vi "wechatSuperResolutionCoffeeModel.vi"() -> (0 "Model":string, 1 "ProtoTxt":string)   [LabVIEW 2020]
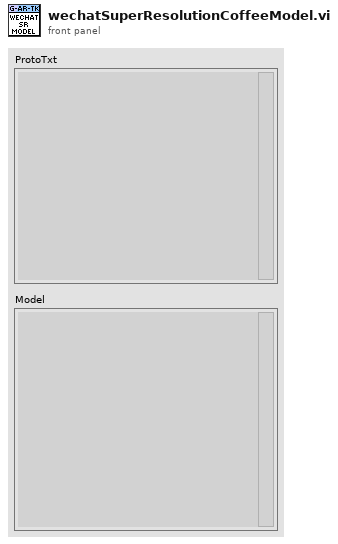
[diagram p1: front panel]
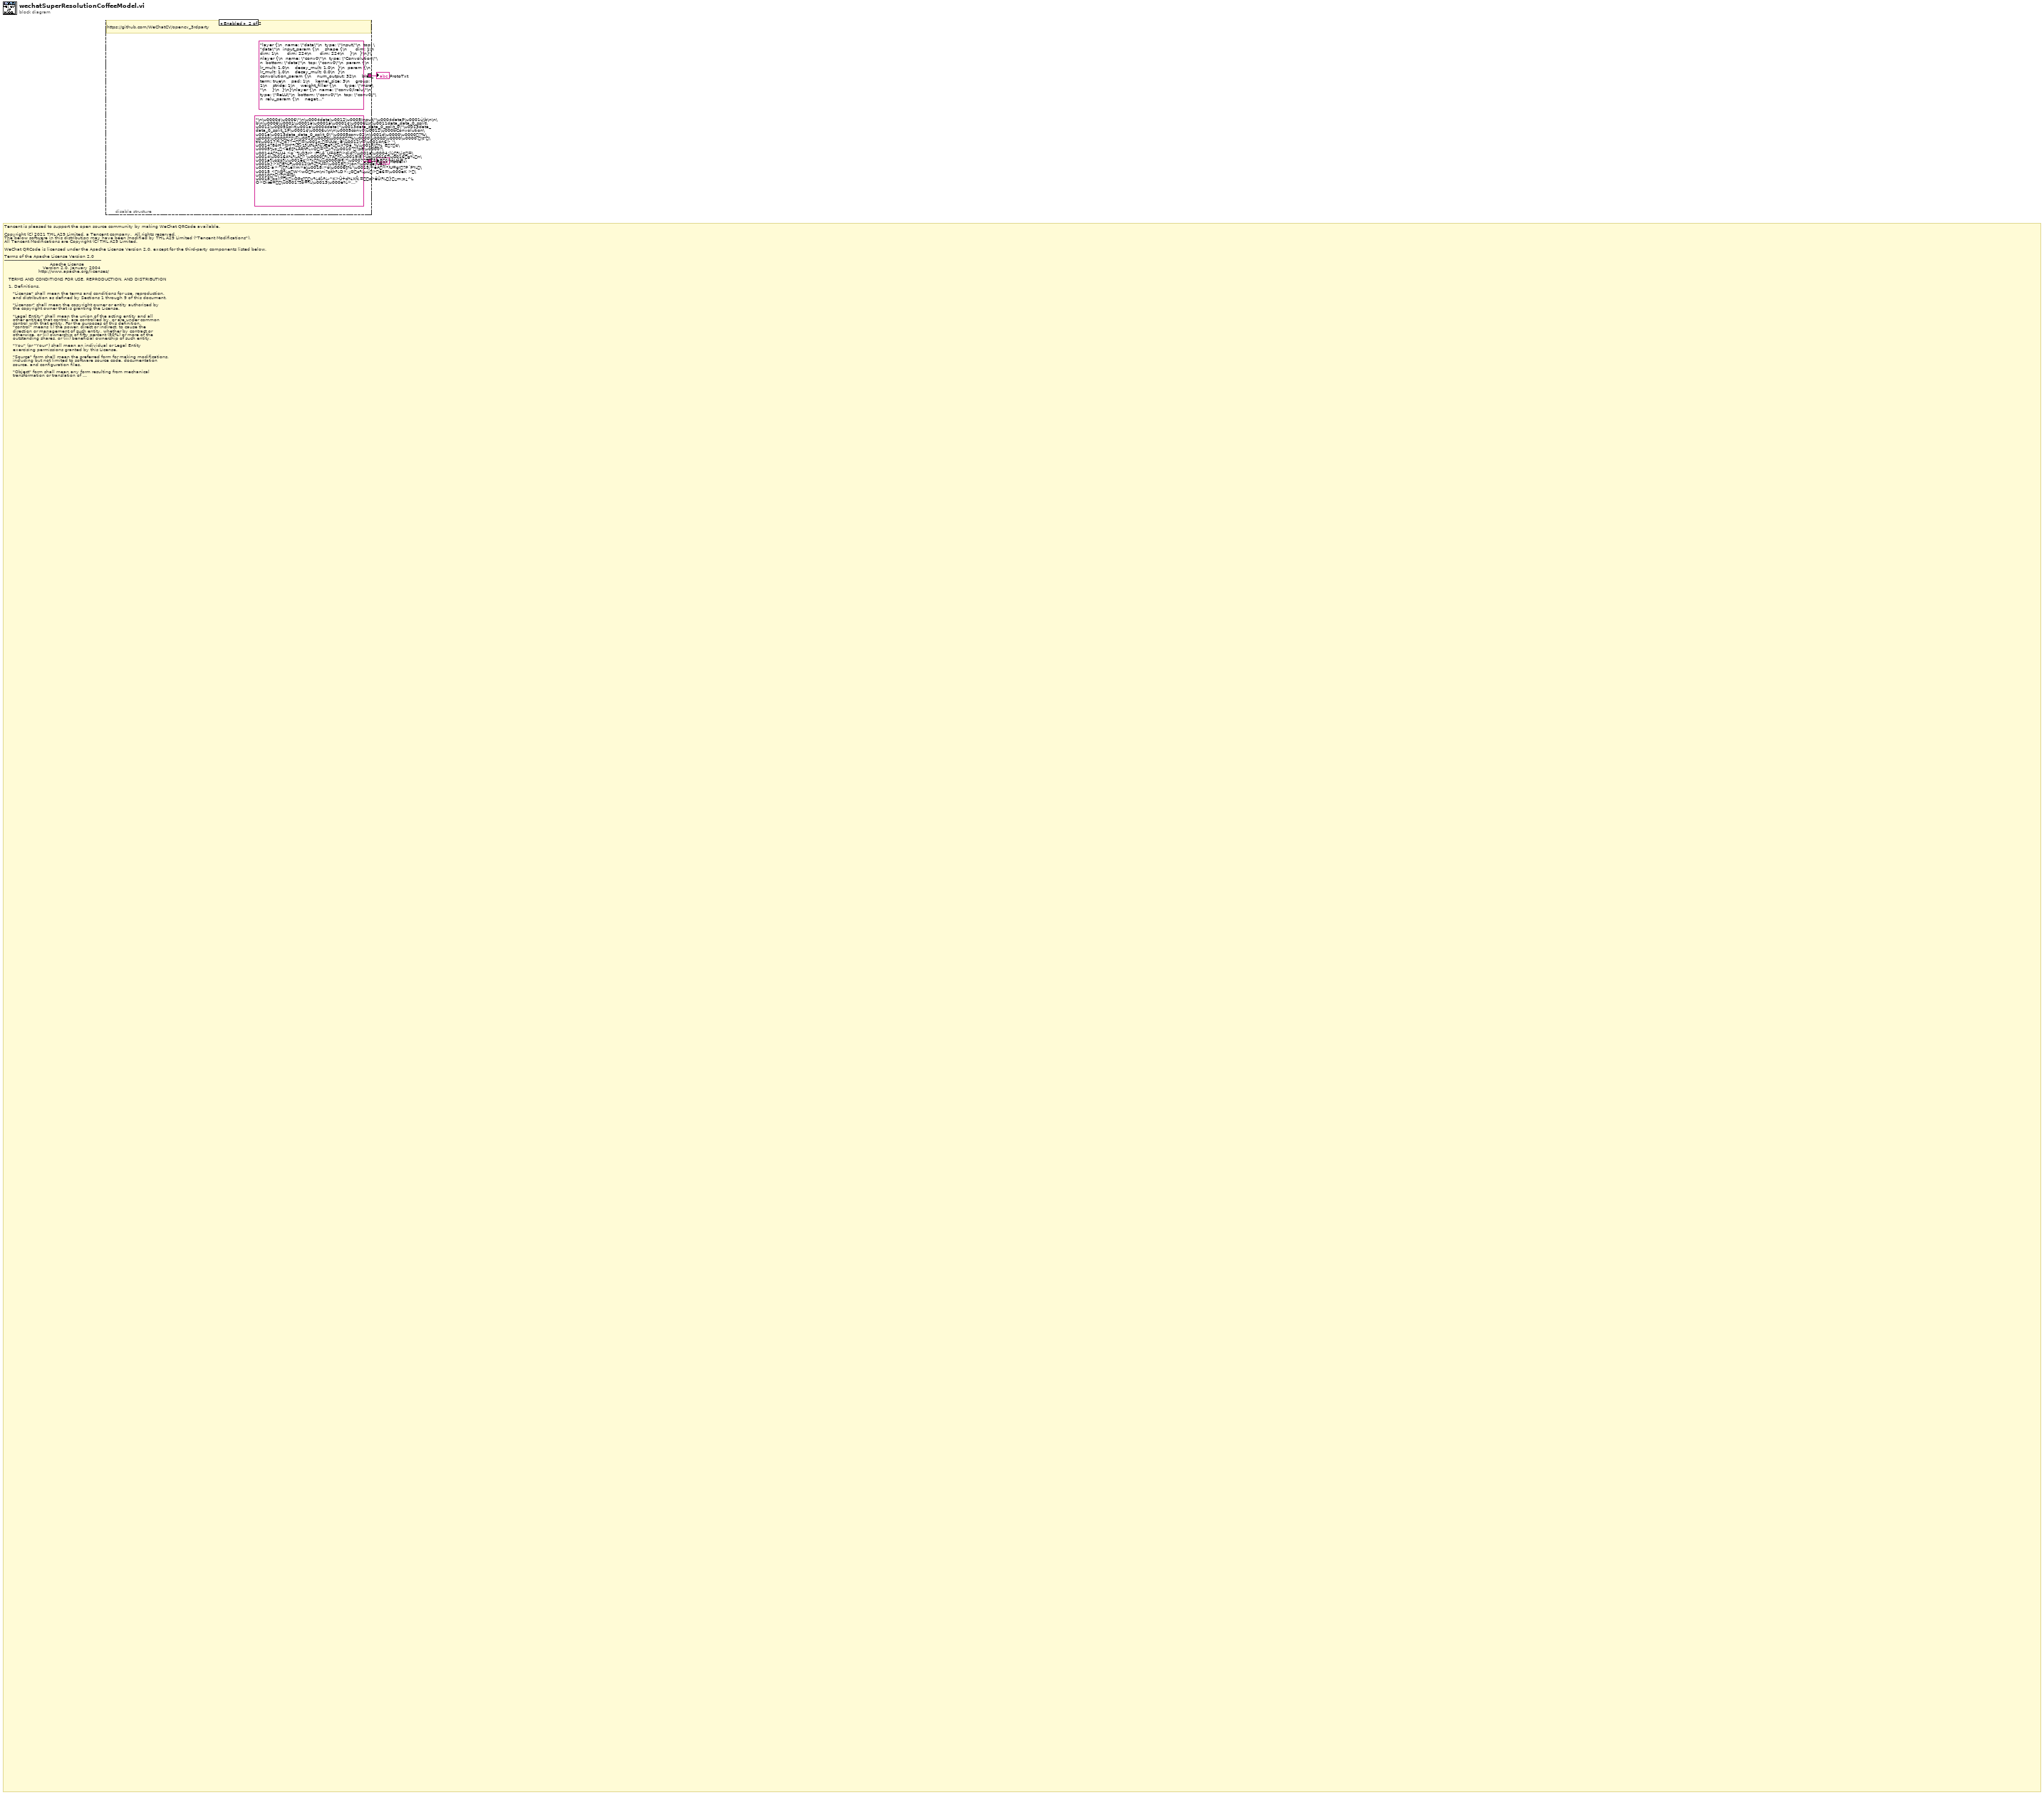
[diagram p0: block diagram]
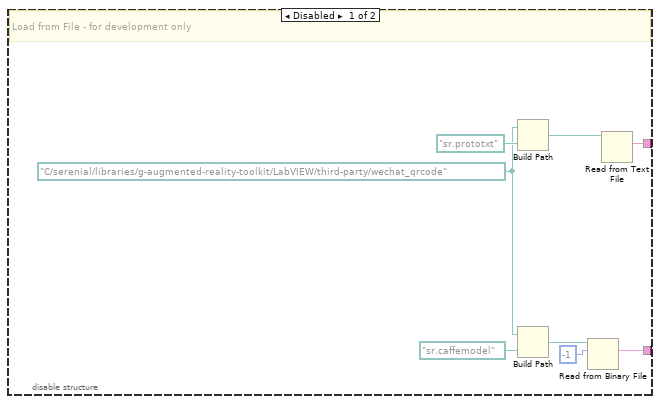
[diagram p2: hidden frame]
diagram:
  # "Tencent is pleased to support the open source community by making WeChat QRCode available.\n\nCopyright (C) 2021 THL A29 Limited, a Tencent company.  All rights reserved.\nThe below software in this distribution may have been modified by THL A29 Limited (\"Tencent Modifications\").\nAll Tencent Modifications are Copyright (C) THL A29 Limited.\n\nWeChat QRCode is licensed under the Apache License Version 2.0, except for the third-party components listed below.\n\nTerms of the Apache License Version 2.0\n--------------------------------------------------------------------\n                                Apache License\n                           Version 2.0, January 2004\n                        http://www.apache.org/licenses/\n\n   TERMS AND CONDITIONS FOR USE, REPRODUCTION, AND DISTRIBUTION\n\n   1. Definitions.\n\n      \"License\" shall mean the terms and conditions for use, reproduction,\n      and distribution as defined by Sections 1 through 9 of this document.\n\n      \"Licensor\" shall mean the copyright owner or entity authorized by\n      the copyright owner that is granting the License.\n\n      \"Legal Entity\" shall mean the union of the acting entity and all\n      other entities that control, are controlled by, or are under common\n      control with that entity. For the purposes of this definition,\n      \"control\" means (i) the power, direct or indirect, to cause the\n      direction or management of such entity, whether by contract or\n      otherwise, or (ii) ownership of fifty percent (50%) or more of the\n      outstanding shares, or (iii) beneficial ownership of such entity.\n\n      \"You\" (or \"Your\") shall mean an individual or Legal Entity\n      exercising permissions granted by this License.\n\n      \"Source\" form shall mean the preferred form for making modifications,\n      including but not limited to software source code, documentation\n      source, and configuration files.\n\n      \"Object\" form shall mean any form resulting from mechanical\n      transformation or translation of a Source form, including but\n      not limited to compiled object code, generated documentation,\n      and conversions to other media types.\n\n      \"Work\" shall mean the work of authorship, whether in Source or\n      Object form, made available under the License, as indicated by a\n      copyright notice that is included in or attached to the work\n      (an example is provided in the Appendix below).\n\n      \"Derivative Works\" shall mean any work, whether in Source or Object\n      form, that is based on (or derived from) the Work and for which the\n      editorial revisions, annotations, elaborations, or other modifications\n      represent, as a whole, an original work of authorship. For the purposes\n      of this License, Derivative Works shall not include works that remain\n      separable from, or merely link (or bind by name) to the interfaces of,\n      the Work and Derivative Works thereof.\n\n      \"Contribution\" shall mean any work of authorship, including\n      the original version of the Work and any modifications or additions\n      to that Work or Derivative Works thereof, that is intentionally\n      submitted to Licensor for inclusion in the Work by the copyright owner\n      or by an individual or Legal Entity authorized to submit on behalf of\n      the copyright owner. For the purposes of this definition, \"submitted\"\n      means any form of electronic, verbal, or written communication sent\n      to the Licensor or its representatives, including but not limited to\n      communication on electronic mailing lists, source code control systems,\n      and issue tracking systems that are managed by, or on behalf of, the\n      Licensor for the purpose of discussing and improving the Work, but\n      excluding communication that is conspicuously marked or otherwise\n      designated in writing by the copyright owner as \"Not a Contribution.\"\n\n      \"Contributor\" shall mean Licensor and any individual or Legal Entity\n      on behalf of whom a Contribution has been received by Licensor and\n      subsequently incorporated within the Work.\n\n   2. Grant of Copyright License. Subject to the terms and conditions of\n      this License, each Contributor hereby grants to You a perpetual,\n      worldwide, non-exclusive, no-charge, royalty-free, irrevocable\n      copyright license to reproduce, prepare Derivative Works of,\n      publicly display, publicly perform, sublicense, and distribute the\n      Work and such Derivative Works in Source or Object form.\n\n   3. Grant of Patent License. Subject to the terms and conditions of\n      this License, each Contributor hereby grants to You a perpetual,\n      worldwide, non-exclusive, no-charge, royalty-free, irrevocable\n      (except as stated in this section) patent license to make, have made,\n      use, offer to sell, sell, import, and otherwise transfer the Work,\n      where such license applies only to those patent claims licensable\n      by such Contributor that are necessarily infringed by their\n      Contribution(s) alone or by combination of their Contribution(s)\n      with the Work to which such Contribution(s) was submitted. If You\n      institute patent litigation against any entity (including a\n      cross-claim or counterclaim in a lawsuit) alleging that the Work\n      or a Contribution incorporated within the Work constitutes direct\n      or contributory patent infringement, then any patent licenses\n      granted to You under this License for that Work shall terminate\n      as of the date such litigation is filed.\n\n   4. Redistribution. You may reproduce and distribute copies of the\n      Work or Derivative Works thereof in any medium, with or without\n      modifications, and in Source or Object form, provided that You\n      meet the following conditions:\n\n      (a) You must give any other recipients of the Work or\n          Derivative Works a copy of this License; and\n\n      (b) You must cause any modified files to carry prominent notices\n          stating that You changed the files; and\n\n      (c) You must retain, in the Source form of any Derivative Works\n          that You distribute, all copyright, patent, trademark, and\n          attribution notices from the Source form of the Work,\n          excluding those notices that do not pertain to any part of\n          the Derivative Works; and\n\n      (d) If the Work includes a \"NOTICE\" text file as part of its\n          distribution, then any Derivative Works that You distribute must\n          include a readable copy of the attribution notices contained\n          within such NOTICE file, excluding those notices that do not\n          pertain to any part of the Derivative Works, in at least one\n          of the following places: within a NOTICE text file distributed\n          as part of the Derivative Works; within the Source form or\n          documentation, if provided along with the Derivative Works; or,\n          within a display generated by the Derivative Works, if and\n          wherever such third-party notices normally appear. The contents\n          of the NOTICE file are for informational purposes only and\n          do not modify the License. You may add Your own attribution\n          notices within Derivative Works that You distribute, alongside\n          or as an addendum to the NOTICE text from the Work, provided\n          that such additional attribution notices cannot be construed\n          as modifying the License.\n\n      You may add Your own copyright statement to Your modifications and\n      may provide additional or different license terms and conditions\n      for use, reproduction, or distribution of Your modifications, or\n      for any such Derivative Works as a whole, provided Your use,\n      reproduction, and distribution of the Work otherwise complies with\n      the conditions stated in this License.\n\n   5. Submission of Contributions. Unless You explicitly state otherwise,\n      any Contribution intentionally submitted for inclusion in the Work\n      by You to the Licensor shall be under the terms and conditions of\n      this License, without any additional terms or conditions.\n      Notwithstanding the above, nothing herein shall supersede or modify\n      the terms of any separate license agreement you may have executed\n      with Licensor regarding such Contributions.\n\n   6. Trademarks. This License does not grant permission to use the trade\n      names, trademarks, service marks, or product names of the Licensor,\n      except as required for reasonable and customary use in describing the\n      origin of the Work and reproducing the content of the NOTICE file.\n\n   7. Disclaimer of Warranty. Unless required by applicable law or\n      agreed to in writing, Licensor provides the Work (and each\n      Contributor provides its Contributions) on an \"AS IS\" BASIS,\n      WITHOUT WARRANTIES OR CONDITIONS OF ANY KIND, either express or\n      implied, including, without limitation, any warranties or conditions\n      of TITLE, NON-INFRINGEMENT, MERCHANTABILITY, or FITNESS FOR A\n      PARTICULAR PURPOSE. You are solely responsible for determining the\n      appropriateness of using or redistributing the Work and assume any\n      risks associated with Your exercise of permissions under this License.\n\n   8. Limitation of Liability. In no event and under no legal theory,\n      whether in tort (including negligence), contract, or otherwise,\n      unless required by applicable law (such as deliberate and grossly\n      negligent acts) or agreed to in writing, shall any Contributor be\n      liable to You for damages, including any direct, indirect, special,\n      incidental, or consequential damages of any character arising as a\n      result of this License or out of the use or inability to use the\n      Work (including but not limited to damages for loss of goodwill,\n      work stoppage, computer failure or malfunction, or any and all\n      other commercial damages or losses), even if such Contributor\n      has been advised of the possibility of such damages.\n\n   9. Accepting Warranty or Additional Liability. While redistributing\n      the Work or Derivative Works thereof, You may choose to offer,\n      and charge a fee for, acceptance of support, warranty, indemnity,\n      or other liability obligations and/or rights consistent with this\n      License. However, in accepting such obligations, You may act only\n      on Your own behalf and on Your sole responsibility, not on behalf\n      of any other Contributor, and only if You agree to indemnify,\n      defend, and hold each Contributor harmless for any liability\n      incurred by, or claims asserted against, such Contributor by reason\n      of your accepting any such warranty or additional liability.\n\nEND OF TERMS AND CONDITIONS\n\n\n\nOther dependencies and licenses:\n\nOpen Source Software Licensed under the Apache License Version 2.0:\n--------------------------------------------------------------------\n1. zxing\nCopyright (c) zxing authors and contributors\nPlease note this software may have been modified by Tencent.\n\nTerms of the Apache License Version 2.0:\n--------------------------------------------------------------------\nApache License\n\nVersion 2.0, January 2004\n\nhttp://www.apache.org/licenses/\n\nTERMS AND CONDITIONS FOR USE, REPRODUCTION, AND DISTRIBUTION\n\n1. Definitions.\n\n\"License\" shall mean the terms and conditions for use, reproduction, and distribution as defined by Sections 1 through 9 of this document.\n\n\"Licensor\" shall mean the copyright owner or entity authorized by the copyright owner that is granting the License.\n\n\"Legal Entity\" shall mean the union of the acting entity and all other entities that control, are controlled by, or are under common control with that entity. For the purposes of this definition, \"control\" means (i) the power, direct or indirect, to cause the direction or management of such entity, whether by contract or otherwise, or (ii) ownership of fifty percent (50%) or more of the outstanding shares, or (iii) beneficial ownership of such entity.\n\n\"You\" (or \"Your\") shall mean an individual or Legal Entity exercising permissions granted by this License.\n\n\"Source\" form shall mean the preferred form for making modifications, including but not limited to software source code, documentation source, and configuration files.\n\n\"Object\" form shall mean any form resulting from mechanical transformation or translation of a Source form, including but not limited to compiled object code, generated documentation, and conversions to other media types.\n\n\"Work\" shall mean the work of authorship, whether in Source or Object form, made available under the License, as indicated by a copyright notice that is included in or attached to the work (an example is provided in the Appendix below).\n\n\"Derivative Works\" shall mean any work, whether in Source or Object form, that is based on (or derived from) the Work and for which the editorial revisions, annotations, elaborations, or other modifications represent, as a whole, an original work of authorship. For the purposes of this License, Derivative Works shall not include works that remain separable from, or merely link (or bind by name) to the interfaces of, the Work and Derivative Works thereof.\n\n\"Contribution\" shall mean any work of authorship, including the original version of the Work and any modifications or additions to that Work or Derivative Works thereof, that is intentionally submitted to Licensor for inclusion in the Work by the copyright owner or by an individual or Legal Entity authorized to submit on behalf of the copyright owner. For the purposes of this definition, \"submitted\" means any form of electronic, verbal, or written communication sent to the Licensor or its representatives, including but not limited to communication on electronic mailing lists, source code control systems, and issue tracking systems that are managed by, or on behalf of, the Licensor for the purpose of discussing and improving the Work, but excluding communication that is conspicuously marked or otherwise designated in writing by the copyright owner as \"Not a Contribution.\"\n\n\"Contributor\" shall mean Licensor and any individual or Legal Entity on behalf of whom a Contribution has been received by Licensor and subsequently incorporated within the Work.\n\n2. Grant of Copyright License. Subject to the terms and conditions of this License, each Contributor hereby grants to You a perpetual, worldwide, non-exclusive, no-charge, royalty-free, irrevocable copyright license to reproduce, prepare Derivative Works of, publicly display, publicly perform, sublicense, and distribute the Work and such Derivative Works in Source or Object form.\n\n3. Grant of Patent License. Subject to the terms and conditions of this License, each Contributor hereby grants to You a perpetual, worldwide, non-exclusive, no-charge, royalty-free, irrevocable (except as stated in this section) patent license to make, have made, use, offer to sell, sell, import, and otherwise transfer the Work, where such license applies only to those patent claims licensable by such Contributor that are necessarily infringed by their Contribution(s) alone or by combination of their Contribution(s) with the Work to which such Contribution(s) was submitted. If You institute patent litigation against any entity (including a cross-claim or counterclaim in a lawsuit) alleging that the Work or a Contribution incorporated within the Work constitutes direct or contributory patent infringement, then any patent licenses granted to You under this License for that Work shall terminate as of the date such litigation is filed.\n\n4. Redistribution. You may reproduce and distribute copies of the Work or Derivative Works thereof in any medium, with or without modifications, and in Source or Object form, provided that You meet the following conditions:\n\nYou must give any other recipients of the Work or Derivative Works a copy of this License; and\nYou must cause any modified files to carry prominent notices stating that You changed the files; and\nYou must retain, in the Source form of any Derivative Works that You distribute, all copyright, patent, trademark, and attribution notices from the Source form of the Work, excluding those notices that do not pertain to any part of the Derivative Works; and\nIf the Work includes a \"NOTICE\" text file as part of its distribution, then any Derivative Works that You distribute must include a readable copy of the attribution notices contained within such NOTICE file, excluding those notices that do not pertain to any part of the Derivative Works, in at least one of the following places: within a NOTICE text file distributed as part of the Derivative Works; within the Source form or documentation, if provided along with the Derivative Works; or, within a display generated by the Derivative Works, if and wherever such third-party notices normally appear. The contents of the NOTICE file are for informational purposes only and do not modify the License. You may add Your own attribution notices within Derivative Works that You distribute, alongside or as an addendum to the NOTICE text from the Work, provided that such additional attribution notices cannot be construed as modifying the License.\n\nYou may add Your own copyright statement to Your modifications and may provide additional or different license terms and conditions for use, reproduction, or distribution of Your modifications, or for any such Derivative Works as a whole, provided Your use, reproduction, and distribution of the Work otherwise complies with the conditions stated in this License.\n\n5. Submission of Contributions. Unless You explicitly state otherwise, any Contribution intentionally submitted for inclusion in the Work by You to the Licensor shall be under the terms and conditions of this License, without any additional terms or conditions. Notwithstanding the above, nothing herein shall supersede or modify the terms of any separate license agreement you may have executed with Licensor regarding such Contributions.\n\n6. Trademarks. This License does not grant permission to use the trade names, trademarks, service marks, or product names of the Licensor, except as required for reasonable and customary use in describing the origin of the Work and reproducing the content of the NOTICE file.\n\n7. Disclaimer of Warranty. Unless required by applicable law or agreed to in writing, Licensor provides the Work (and each Contributor provides its Contributions) on an \"AS IS\" BASIS, WITHOUT WARRANTIES OR CONDITIONS OF ANY KIND, either express or implied, including, without limitation, any warranties or conditions of TITLE, NON-INFRINGEMENT, MERCHANTABILITY, or FITNESS FOR A PARTICULAR PURPOSE. You are solely responsible for determining the appropriateness of using or redistributing the Work and assume any risks associated with Your exercise of permissions under this License.\n\n8. Limitation of Liability. In no event and under no legal theory, whether in tort (including negligence), contract, or otherwise, unless required by applicable law (such as deliberate and grossly negligent acts) or agreed to in writing, shall any Contributor be liable to You for damages, including any direct, indirect, special, incidental, or consequential damages of any character arising as a result of this License or out of the use or inability to use the Work (including but not limited to damages for loss of goodwill, work stoppage, computer failure or malfunction, or any and all other commercial damages or losses), even if such Contributor has been advised of the possibility of such damages.\n\n9. Accepting Warranty or Additional Liability. While redistributing the Work or Derivative Works thereof, You may choose to offer, and charge a fee for, acceptance of support, warranty, indemnity, or other liability obligations and/or rights consistent with this License. However, in accepting such obligations, You may act only on Your own behalf and on Your sole responsibility, not on behalf of any other Contributor, and only if You agree to indemnify, defend, and hold each Contributor harmless for any liability incurred by, or claims asserted against, such Contributor by reason of your accepting any such warranty or additional liability.\n\nEND OF TERMS AND CONDITIONS"
  n1 = disable-structure shown="Enabled" {
    disable-tunnel: [w5 "\n\u0000¢\u0006\"\n\u0004data\u0012\u0005Input\"\u0004dataP\u0001ú\b\n\n\b\n\u0006\u0001\u0001à\u0001à\u0001¢\u0006L\n\u0011data_data_0_split\u0012\u0005Split\u001a\u0004data\"\u0013data_data_0_split_0\"\u0013data_data_0_split_1P\u0001¢\u0006ú\n\n\u0005conv0\u0012\u000bConvolution\u001a\u0013data_data_0_split_0\"\u0005conv02\n\u001d\u0000\u0000?%\u0000\u0000?2\n\u001d\u0000\u0000?%\u0000\u0000\u0000\u0000:\t*\tÑ\u0017|¾ö7?¬=\u001c¿=ÜÙ¥¿©\u0012\r=\u0014ñ6>´'\u0014?8òH>§M*¾ºv1¾t%Å½:Æe¾ùX?Öâ¸½\u001f\\½´Ê?¢\u0005½¤¿<é£§½ÅRÑ¾»Ò=*«¾\u0010¯?pB\u0000?\u0014Ä½Ú4 <ø`'¾Ò3r> :F¾ö`Ü=ôÊ>did?ï\u001a\u0004¿lù¾i¢=\u0014\u0016À½¾Ã? \u0000¾TA¼\u0019ÎÊ>Ûq\u0016?\u0016g¼n\u001a¾q¥¤¾\u001eç!>²x½\u0000@¶:*\u0007¾$¦¿8§>ñÜñ=¿\u001b}>XÈ½F\u0012\b¾¹Ú=ï\u0015>Jôn?\u001e\"Æ¿\u0002·á>^J¾éÝm>a\u0018:>ø\u0006§½'\u0015/>èÄ<°)U=gI?P´P¼\u0015 <I@¾pW<wÕ¾m\ni?çÁh¾D×;¿Øø¾µû>ë6=\u000eK >\u0010½\"=lþ\u0018¿b¤)>K»OPç?v¾4[-¾­^K>Ü+d½XÑ,=s>ëÛ!¾}¿m¡¤¿^LÔ>Dìæ=\u0001?ªö=¾\u0013\u000e¼>..." ("Model")] -> w2
    disable-tunnel: [w3 "layer {\n  name: \"data\"\n  type: \"Input\"\n  top: \"data\"\n  input_param {\n    shape {\n      dim: 1\n      dim: 1\n      dim: 224\n      dim: 224\n    }\n  }\n}\nlayer {\n  name: \"conv0\"\n  type: \"Convolution\"\n  bottom: \"data\"\n  top: \"conv0\"\n  param {\n    lr_mult: 1.0\n    decay_mult: 1.0\n  }\n  param {\n    lr_mult: 1.0\n    decay_mult: 0.0\n  }\n  convolution_param {\n    num_output: 32\n    bias_term: true\n    pad: 1\n    kernel_size: 3\n    group: 1\n    stride: 1\n    weight_filler {\n      type: \"msra\"\n    }\n  }\n}\nlayer {\n  name: \"conv0/lrelu\"\n  type: \"ReLU\"\n  bottom: \"conv0\"\n  top: \"conv0\"\n  relu_param {\n    negative_slope: 0.05000000074505806\n  }\n}\nlayer {\n  name: \"db1/reduce\"\n  type: \"Convolution\"\n  bottom: \"conv0\"\n  top: \"db1/reduce\"\n  param {\n    lr_mult: 1.0\n    decay_mult: 1.0\n  }\n  param {\n    lr_mult: 1.0\n    decay_mult: 0.0\n  }\n  convolution_param {\n    num_output: 8\n    bias_term: true\n    pad: 0\n    kernel_size: 1\n    group: 1\n    stride: 1\n    weight_filler {\n      type: \"msra\"\n    }\n  }\n}\nlayer {\n  name: \"db1/reduce/lrelu\"\n  type: \"ReLU\"\n  bottom: \"db1/reduce\"\n  top: \"db1/reduce\"\n  relu_param {\n    negative_slope: 0.05000000074505806\n  }\n}\nlayer {\n  name: \"db1/3x3\"\n  type: \"Convolution\"\n  bottom: \"db1/reduce\"\n  top: \"db1/3x3\"\n  param {\n    lr_mult: 1.0\n    decay_mult: 1.0\n  }\n  param {\n    lr_mult: 1.0\n    decay_mult: 0.0\n  }\n  convolution_param {\n    num_output: 8\n    bias_term: true\n    pad: 1\n    kernel_size: 3\n    group: 8\n    stride: 1\n    weight_filler {\n      type: \"msra\"\n    }\n  }\n}\nlayer {\n  name: \"db1/3x3/lrelu\"\n  type: \"ReLU\"\n  bottom: \"db1/3x3\"\n  top: \"db1/3x3\"\n  relu_param {\n    negative_slope: 0.05000000074505806\n  }\n}\nlayer {\n  name: \"db1/1x1\"\n  type: \"Convolution\"\n  bottom: \"db1/3x3\"\n  top: \"db1/1x1\"\n  param {\n    lr_mult: 1.0\n    decay_mult: 1.0\n  }\n  param {\n    lr_mult: 1.0\n    decay_mult: 0.0\n  }\n  convolution_param {\n    num_output: 32\n    bias_term: true\n    pad: 0\n    kernel_size: 1\n    group: 1\n    stride: 1\n    weight_filler {\n      type: \"msra\"\n    }\n  }\n}\nlayer {\n  name: \"db1/1x1/lrelu\"\n  type: \"ReLU\"\n  bottom: \"db1/1x1\"\n  top: \"db1/1x1\"\n  relu_param {\n    negative_slope: 0.05000000074505806\n  }\n}\nlayer {\n  name: \"db1/concat\"\n  type: \"Concat\"\n  bottom: \"conv0\"\n  bottom: \"db1/1x1\"\n  top: \"db1/concat\"\n  concat_param {\n    axis: 1\n  }\n}\nlayer {\n  name: \"db2/reduce\"\n  type: \"Convolution\"\n  bottom: \"db1/concat\"\n  top: \"db2/reduce\"\n  param {\n    lr_mult: 1.0\n    decay_mult: 1.0\n  }\n  param {\n    lr_mult: 1.0\n    decay_mult: 0.0\n  }\n  convolution_param {\n    num_output: 8\n    bias_term: true\n    pad: 0\n    kernel_size: 1\n    group: 1\n    stride: 1\n    weight_filler {\n      type: \"msra\"\n    }\n  }\n}\nlayer {\n  name: \"db2/reduce/lrelu\"\n  type: \"ReLU\"\n  bottom: \"db2/reduce\"\n  top: \"db2/reduce\"\n  relu_param {\n    negative_slope: 0.05000000074505806\n  }\n}\nlayer {\n  name: \"db2/3x3\"\n  type: \"Convolution\"\n  bottom: \"db2/reduce\"\n  top: \"db2/3x3\"\n  param {\n    lr_mult: 1.0\n    decay_mult: 1.0\n  }\n  param {\n    lr_mult: 1.0\n    decay_mult: 0.0\n  }\n  convolution_param {\n    num_output: 8\n    bias_term: true\n    pad: 1\n    kernel_size: 3\n    group: 8\n    stride: 1\n    weight_filler {\n      type: \"msra\"\n    }\n  }\n}\nlayer {\n  name: \"db2/3x3/lrelu\"\n  type: \"ReLU\"\n  bottom: \"db2/3x3\"\n  top: \"db2/3x3\"\n  relu_param {\n    negative_slope: 0.05000000074505806\n  }\n}\nlayer {\n  name: \"db2/1x1\"\n  type: \"Convolution\"\n  bottom: \"db2/3x3\"\n  top: \"db2/1x1\"\n  param {\n    lr_mult: 1.0\n    decay_mult: 1.0\n  }\n  param {\n    lr_mult: 1.0\n    decay_mult: 0.0\n  }\n  convolution_param {\n    num_output: 32\n    bias_term: true\n    pad: 0\n    kernel_size: 1\n    group: 1\n    stride: 1\n    weight_filler {\n      type: \"msra\"\n    }\n  }\n}\nlayer {\n  name: \"db2/1x1/lrelu\"\n  type: \"ReLU\"\n  bottom: \"db2/1x1\"\n  top: \"db2/1x1\"\n  relu_param {\n    negative_slope: 0.05000000074505806\n  }\n}\nlayer {\n  name: \"db2/concat\"\n  type: \"Concat\"\n  bottom: \"db1/concat\"\n  bottom: \"db2/1x1\"\n  top: \"db2/concat\"\n  concat_param {\n    axis: 1\n  }\n}\nlayer {\n  name: \"upsample/reduce\"\n  type: \"Convolution\"\n  bottom: \"db2/concat\"\n  top: \"upsample/reduce\"\n  param {\n    lr_mult: 1.0\n    decay_mult: 1.0\n  }\n  param {\n    lr_mult: 1.0\n    decay_mult: 0.0\n  }\n  convolution_param {\n    num_output: 32\n    bias_term: true\n    pad: 0\n    kernel_size: 1\n    group: 1\n    stride: 1\n    weight_filler {\n      type: \"msra\"\n    }\n  }\n}\nlayer {\n  name: \"upsample/reduce/lrelu\"\n  type: \"ReLU\"\n  bottom: \"upsample/reduce\"\n  top: \"upsample/reduce\"\n  relu_param {\n    negative_slope: 0.05000000074505806\n  }\n}\nlayer {\n  name: \"upsample/deconv\"\n  type: \"Deconvolution\"\n  bottom: \"upsample/reduce\"\n  top: \"upsample/deconv\"\n  param {\n    lr_mult: 1.0\n    decay_mult: 1.0\n  }\n  param {\n    lr_mult: 1.0\n    decay_mult: 0.0\n  }\n  convolution_param {\n    num_output: 32\n    bias_term: true\n    pad: 1\n    kernel_size: 3\n    group: 32\n    stride: 2\n    weight_filler {\n      type: \"msra\"\n    }\n  }\n}\nlayer {\n  name: \"upsample/lrelu\"\n  type: \"ReLU\"\n  bottom: \"upsample/deconv\"\n  top: \"upsample/deconv\"\n  relu_param {\n    negative_slope: 0.05000000074505806\n  }\n}\nlayer {\n  name: \"upsample/rec\"\n  type: \"Convolution\"\n  bottom: \"upsample/deconv\"\n  top: \"upsample/rec\"\n  param {\n    lr_mult: 1.0\n    decay_mult: 1.0\n  }\n  param {\n    lr_mult: 1.0\n    decay_mult: 0.0\n  }\n  convolution_param {\n    num_output: 1\n    bias_term: true\n    pad: 0\n    kernel_size: 1\n    group: 1\n    stride: 1\n    weight_filler {\n      type: \"msra\"\n    }\n  }\n}\nlayer {\n  name: \"nearest\"\n  type: \"Deconvolution\"\n  bottom: \"data\"\n  top: \"nearest\"\n  param {\n    lr_mult: 0.0\n    decay_mult: 0.0\n  }\n  convolution_param {\n    num_output: 1\n    bias_term: false\n    pad: 0\n    kernel_size: 2\n    group: 1\n    stride: 2\n    weight_filler {\n      type: \"constant\"\n      value: 1.0\n    }\n  }\n}\nlayer {\n  name: \"Crop1\"\n  type: \"Crop\"\n  bottom: \"nearest\"\n  bottom: \"upsample/rec\"\n  top: \"Crop1\"\n}\nlayer {\n  name: \"fc\"\n  type: \"Eltwise\"\n  bottom: \"Crop1\"\n  bottom: \"upsample/rec\"\n  top: \"fc\"\n  eltwise_param {\n    operation: SUM\n  }\n}\n" ("ProtoTxt")] -> w1
    frame Disabled {
      w7 = path "C:/serenial/libraries/g-augmented-reality-toolkit/LabVIEW/third-party/wechat_qrcode" ("base path")
      # "Load from File - for development only"
      n2 = Build Path(base path=w7, name or relative path=path "sr.prototxt" ("Filepath")) -> (appended path=w4:path)
      n3 = Build Path(base path=w7, name or relative path=path "sr.caffemodel" ("Filepath")) -> (appended path=w6:path)
      n4 = Read from Binary File(10:-1 ("count (1)"), 11:w6) -> (2:w5:string)  [unwired: 4 in, 3 out]
      n5 = Read from Text File(file (use dialog)=w4) -> (text=w3:string)  [unwired: 3 in, 3 out]
    }
    frame Enabled {
      # "https://github.com/WeChatCV/opencv_3rdparty"
    }
  }
  "Model" <- w2
  "ProtoTxt" <- w1
